vi "Control Value to Camera.vi"(4 "error in (no error)":errorcluster, 5 "Tab Control Ref In":T2, 6 "Tree Control In":refnum<vi>, 7 "Attirbutes":T1[](array[typedef])) -> (0 "error out":errorcluster, 3 "Attribute Out":T1)   [LabVIEW 2020, in "Camera Settings Dialog UI.lvlib" / "Camera Settings Dialog.lvclass"]
doc: "The Flush Control Value subVI reads the value of the control, and then sets the value of the attribute in the IMAQdx driver."
uses:
  Camera Settings Dialog.lvclass
  Camera Attribute Info.ctl
  Attribute Type.ctl
panel:
  out "Found?":bool
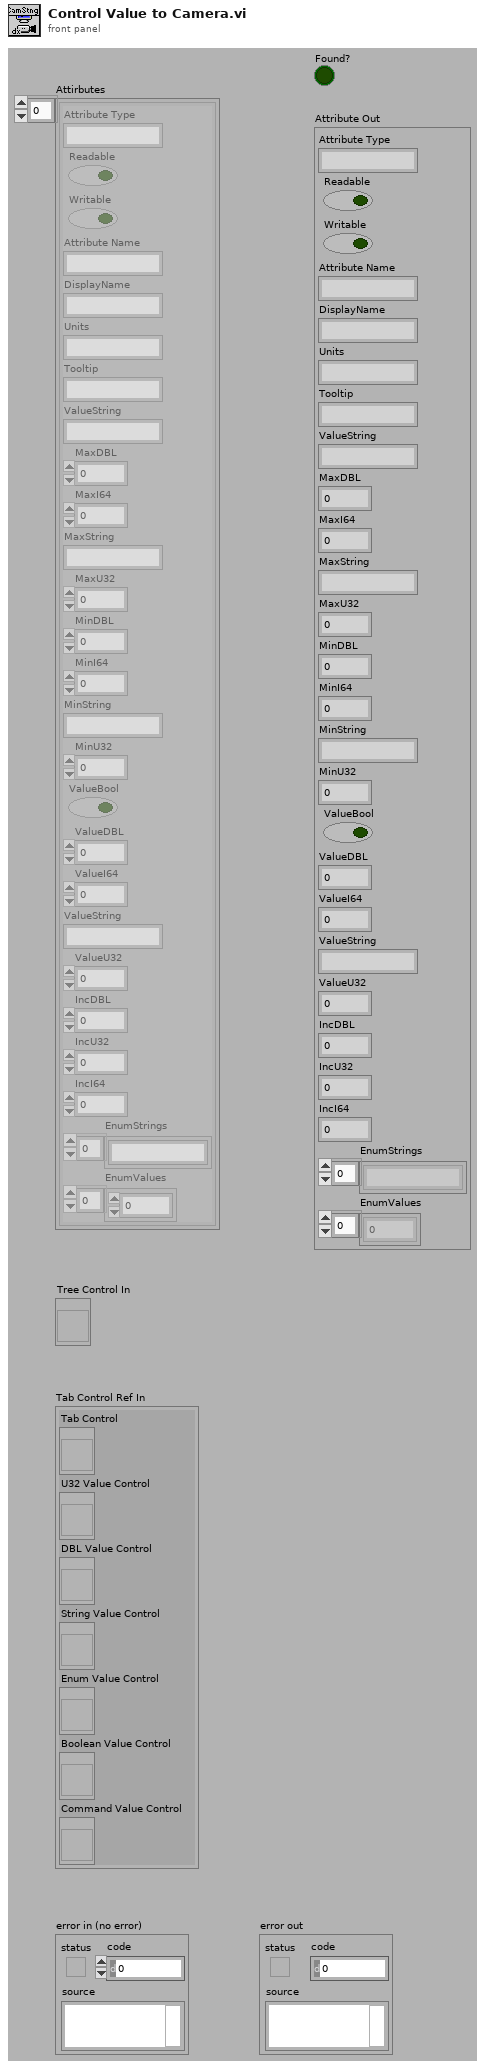
[diagram p1: front panel]
types:
  T1 = typedef "Camera Attribute Info.ctl" = cluster{"Attribute Type":string, "Readable":bool, "Writable":bool, "Attribute Name":string, "DisplayName":string, "Units":string, "Tooltip":string, "ValueString":string, "MaxDBL":dbl, "MaxI64":i64, "MaxString":string, "MaxU32":u32, "MinDBL":dbl, "MinI64":i64, "MinString":string, "MinU32":u32, "ValueBool":bool, "ValueDBL":dbl, "ValueI64 ":i64, "ValueString":string, "ValueU32":u32, "IncDBL":dbl, "IncU32":u32, "IncI64":i64, "EnumStrings":string[], "EnumValues":u32[]}
  T2 = cluster{"Tab Control":refnum<vi>, "U32 Value Control":refnum<vi>, "DBL Value Control":refnum<vi>, "String Value Control":refnum<vi>, "Enum Value Control":refnum<vi>, "Boolean Value Control":refnum<vi>, "Command Value Control":refnum<vi>}
  T3 = typedef "Attribute Type.ctl" = enum32{"U32", "I64", "DBL", "String", "Enum", "Bool", "Command"}
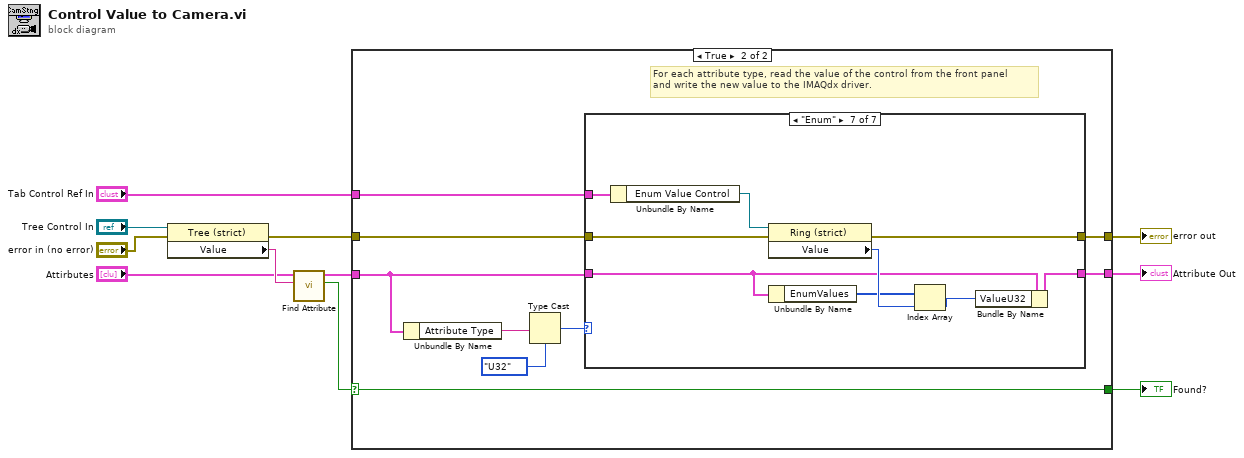
[diagram p0: block diagram]
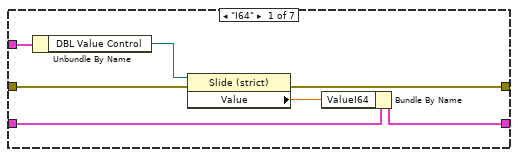
[diagram p3: hidden frame]
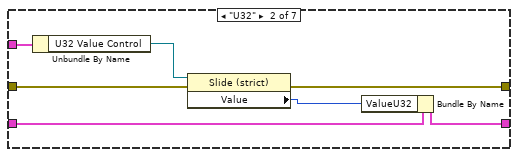
[diagram p4: hidden frame]
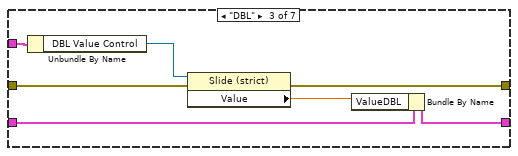
[diagram p5: hidden frame]
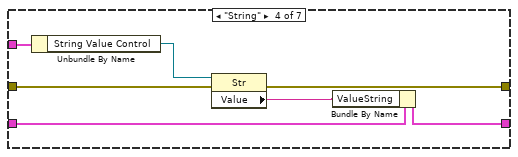
[diagram p6: hidden frame]
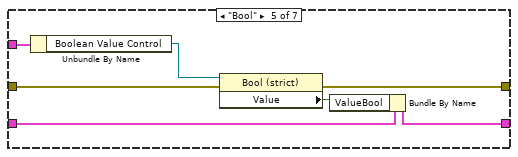
[diagram p7: hidden frame]
diagram:
  n1 = property class="Tree (strict)"(reference="Tree Control In", error in="error in (no error)") -> (error out=w6:errorcluster, "Value"=w7:string)  [unwired: 1 out]
  n2 = call "Find Attribute.vi"("Attr Name"=w7, "Attirbutes"="Attirbutes") -> ("Found?"=w4:bool, "Attribute Information"=w5:T1)  [unwired: 8 in]
  n3 = case shown="True" w4 {
    selector: w4 -> [w12 w15]
    tunnel: "Tab Control Ref In" -> [_ w21]
    tunnel: [w13 w20] -> w8
    tunnel: w6 -> [w13 w19]
    tunnel: w5 -> [w14 w17]
    tunnel: [w14 w16] -> w3
    tunnel: [w12 w15] -> w2
    frame False {
    }
    frame True {
      # "For each attribute type, read the value of the control from the front panel\nand write the new value to the IMAQdx driver."
      n4 = Unbundle By Name(w17) -> ("Attribute Type"=w18:string)
      n5 = Type Cast(type=Attribute_Type."U32" ("Attribute Type"), x=w18) -> (*(type *) &x=w22:T3)
      n6 = case shown="\"Enum\"" w22 {
        tunnel: w19 -> [w28 w35 w42 w49 w56 w60 w67]
        tunnel: w21 -> [w30 w37 w44 w51 w58 _ w69]
        tunnel: [w27 w34 w41 w47 w55 w60 w66] -> w20
        tunnel: w17 -> [w26 w33 w40 w48 w54 w59 w63]
        tunnel: [w25 w32 w39 w46 w53 w59 w62] -> w16
        frame "I64" {
          n7 = Unbundle By Name(w30) -> ("DBL Value Control"=w29:refnum<vi>)
          n8 = property class="Slide (strict)"(reference=w29, error in=w28) -> (error out=w27:errorcluster, "Value"=w24:dbl)  [unwired: 1 out]
          n9 = Bundle By Name(cluster=w26, "ValueI64"=w24) -> (w25:T1)
        }
        frame "U32" {
          n10 = Unbundle By Name(w37) -> ("U32 Value Control"=w36:refnum<vi>)
          n11 = property class="Slide (strict)"(reference=w36, error in=w35) -> (error out=w34:errorcluster, "Value"=w31:u32)  [unwired: 1 out]
          n12 = Bundle By Name(cluster=w33, "ValueU32"=w31) -> (w32:T1)
        }
        frame "DBL" {
          n13 = Unbundle By Name(w44) -> ("DBL Value Control"=w43:refnum<vi>)
          n14 = property class="Slide (strict)"(reference=w43, error in=w42) -> (error out=w41:errorcluster, "Value"=w38:dbl)  [unwired: 1 out]
          n15 = Bundle By Name(cluster=w40, "ValueDBL"=w38) -> (w39:T1)
        }
        frame "String" {
          n16 = Unbundle By Name(w51) -> ("String Value Control"=w50:refnum<vi>)
          n17 = property class="Str"(reference=w50, error in=w49) -> (error out=w47:errorcluster, "Value"=w45:string)  [unwired: 1 out]
          n18 = Bundle By Name(cluster=w48, "ValueString"=w45) -> (w46:T1)
        }
        frame "Bool" {
          n19 = Unbundle By Name(w58) -> ("Boolean Value Control"=w57:refnum<vi>)
          n20 = property class="Bool (strict)"(reference=w57, error in=w56) -> (error out=w55:errorcluster, "Value"=w52:bool)  [unwired: 1 out]
          n21 = Bundle By Name(cluster=w54, "ValueBool"=w52) -> (w53:T1)
        }
        frame "Command" {
        }
        frame "Enum" {
          n22 = Unbundle By Name(w69) -> ("Enum Value Control"=w68:refnum<vi>)
          n23 = property class="Ring (strict)"(reference=w68, error in=w67) -> (error out=w66:errorcluster, "Value"=w65:u32)  [unwired: 1 out]
          n24 = Unbundle By Name(w63) -> ("EnumValues"=w64:u32[])
          n25 = Index Array(array=w64, index=w65) -> (element=w61:u32)
          n26 = Bundle By Name(cluster=w63, "ValueU32"=w61) -> (w62:T1)
        }
      }
    }
  }
  "error out" <- w8
  "Attribute Out" <- w3
  "Found?" <- w2
